vi "usleep.vi"(11 "microseconds":cluster{}) -> ()   [LabVIEW 2019, in "apdm.lvlib"]
doc: "APDM_EXPORT void apdm_usleep(const uint64_t microseconds);"
uses:
  apdm.lvlib
  Lee Lab/CP FES Walking 2018/Code/Working/LabVIEW/apdm.dll
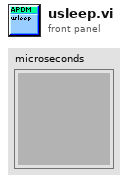
[diagram p1: front panel]
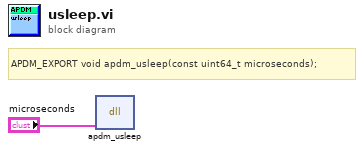
[diagram p0: block diagram]
diagram:
  # "APDM_EXPORT void apdm_usleep(const uint64_t microseconds);"
  n1 = dll-call lib="C:/Users/jfalesi/Dropbox/Lee Lab/CP FES Walking 2018/Code/Working/LabVIEW/apdm.*" fn="apdm_usleep"("microseconds"="microseconds") -> ()  [unwired: 5 in, 2 out]
